vi "pressure_control.vi"() -> ()   [LabVIEW 2018]
uses:
  <vilib>/Analysis/baseanly.llb/Mean (DBL).vi
  <vilib>/addons/control/pid/pid.llb/PID (DBL).vi
  <vilib>/addons/control/pid/NI_PID_pid.lvlib
  <vilib>/Analysis/NI_AALBase.lvlib
panel:
  out "Numeric":i32
  out "mean":dbl=4.714745753355728 format="%0.2f"
  out "subarray":dbl[](array[numeric])
  out "pressure":dbl[][](array[numeric])
  in  "Number of Samples":dbl=10000.0
  in  "Sample Rate [Hz]":dbl=10000.0
  in  "Set control":bool=TRUE
  in  "setpoint":dbl=1.0 format="%.2f"
  in  "PID gains":T1={"proportional gain (Kc)"=1.0, "integral time (Ti, min)"=0.01, "derivative time (Td, min)"=0.0} {"derivative time (Td, min)" format="%.3f"; "integral time (Ti, min)" format="%.3f"; "proportional gain (Kc)" format="%.3f"}
  in  "reinitialize? (F)":bool
  in  "stop":bool
  in  "VISA resource name":refnum<visa-resource-name>="COM3"
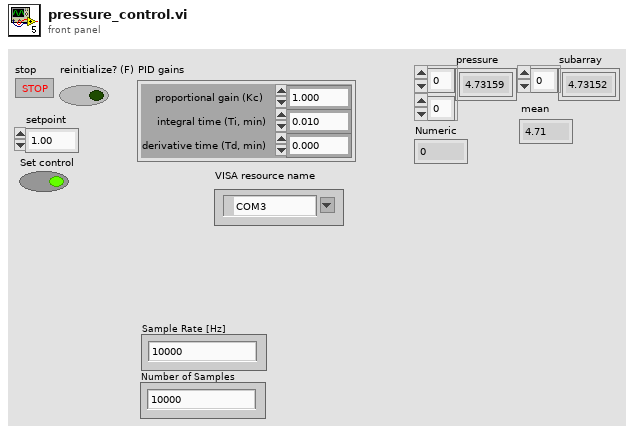
[diagram p1: front panel]
types:
  T1 = cluster{"proportional gain (Kc)":dbl, "integral time (Ti, min)":dbl, "derivative time (Td, min)":dbl}
  T2 = cluster{"Number of Samples":dbl, "Sample Rate [Hz]":dbl, "Physical Channels (Position signals)":tag}
  T3 = cluster{"task out":refnum<k21>, "error out":errorcluster, "SampClk.Rate":dbl}
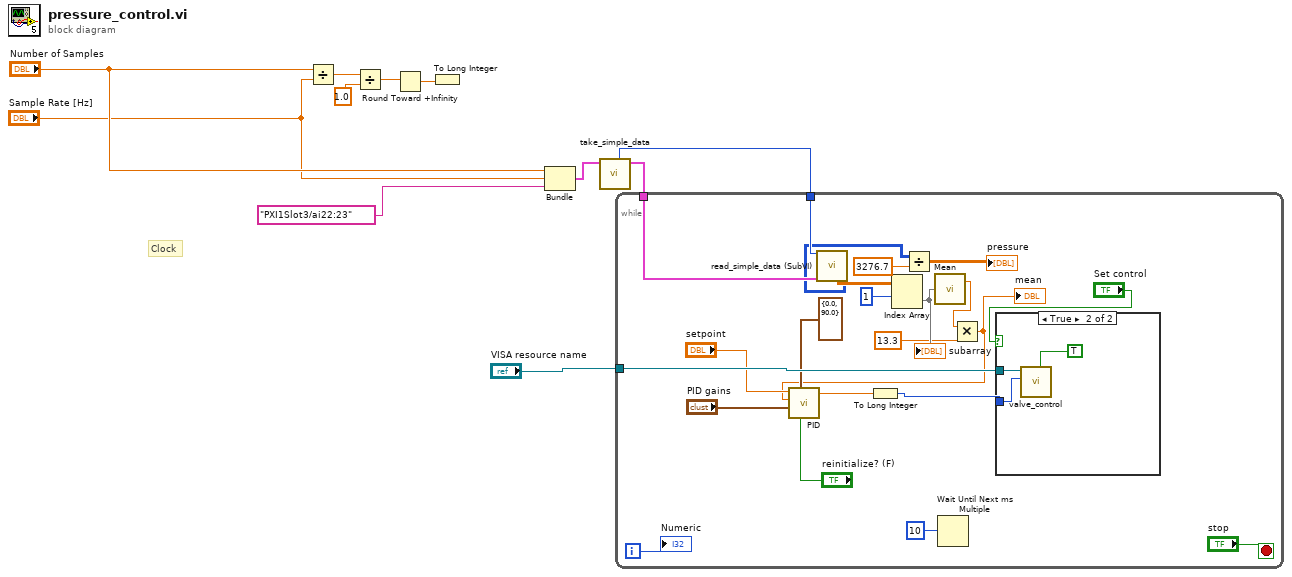
[diagram p0: block diagram]
diagram:
  # "Clock"
  n1 = Divide(x="Number of Samples", y="Sample Rate [Hz]") -> (x/y=w9:dbl)
  n2 = Divide(x=w9, y=1.0) -> (x/y=w7:dbl)
  n3 = Round Toward +Infinity(x=w7) -> (ceil(x): smallest int >= x=w6:dbl)
  n4 = To Long Integer(number=w6) -> ()  [unwired: 1 out]
  n5 = Bundle("Number of Samples"="Number of Samples", "Sample Rate [Hz]"="Sample Rate [Hz]", "Physical Channels (Position signals)"=tag "PXI1Slot3/ai22:23") -> (w3:T2)  [unwired: 1 in]
  n6 = call "take_simple_data.vi"("input cluster"=w3) -> ("number of samples"=w2:i32, "data tasks"=w1:T3)  [unwired: 7 in, 1 out]
  n7 = while {
    tunnel: "VISA resource name" -> [w33]
    tunnel: w2 -> [w24]
    tunnel: w1 -> [w23]
    i -> [w16]
    stop <- "stop" stop-if-true
    n8 = call "read_simple_data (SubVI).vi"("number of samples per channel"=w24, "data tasks"=w23) -> ("data"=w22:dbl[][], "Output data"=w20:i16[][])  [unwired: 10 in, 2 out]
    n9 = Index Array(array=w22, index (row)=1) -> (element=w18:dbl[])  [unwired: 1 in]
    "subarray" <- w18
    n10 = Divide(x=w20, y=3276.7) -> (x/y=→"pressure":dbl[][])
    n11 = call-poly <vilib>:"Mean.vi"("X"=w18) -> ("mean"=w13:dbl)  [unwired: 1 out]
    n12 = Wait Until Next ms Multiple(millisecond multiple=u32 10 ("unsigned 32bit integer")) -> ()  [unwired: 1 out]
    n13 = Multiply(x=w13, y=13.3) -> (x*y=w12:dbl)
    "mean" <- w12
    n14 = call-poly <vilib>:"PID.vi"("reinitialize? (F)"="reinitialize? (F)", "output range"=cluster{"output high":dbl, "output low":dbl} {"output high"=0.0, "output low"=90.0}, "PID gains"="PID gains", "process variable"=w12, "setpoint"="setpoint") -> ("output"=w31:dbl)  [unwired: 5 in, 1 out]
    n15 = To Long Integer(number=w31) -> (32bit integer=w32:i32)
    n16 = case shown="True" "Set control" {
      tunnel: w33 -> [_ w36]
      tunnel: w32 -> [_ w35]
      frame False {
      }
      frame True {
        n17 = call "valve_control.vi"("Set new position"=TRUE, "Valve set pos (deg, 0-90)"=w35, "VISA resource name"=w36) -> ()  [unwired: 8 in, 1 out]
      }
    }
    "Numeric" <- w16
  }
